vi "Display Text from JSON.vi"(5 "No Error on Empty Input String":bool, 7 "Alphabetical Sort Objects":bool, 8 "error in (no error)":errorcluster, 10 "Offset":i32, 11 "Input JSON":string) -> (0 "error out":errorcluster, 1 "Offset after first JSON Value":i32, 3 "Display Text":string)   [LabVIEW 2021, in "json.facade.lvlib"]
doc: "Reformate JSON as a more human-readable text string, for use in displays. The format is similar to YAML, but may not be fully compliant with that format."
uses:
  json.facade.lvlib
  jsontext/JSONtext.lvlib
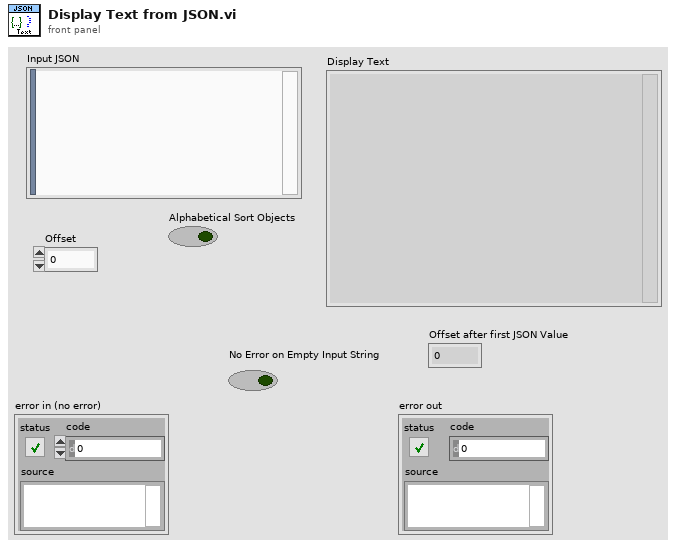
[diagram p1: front panel]
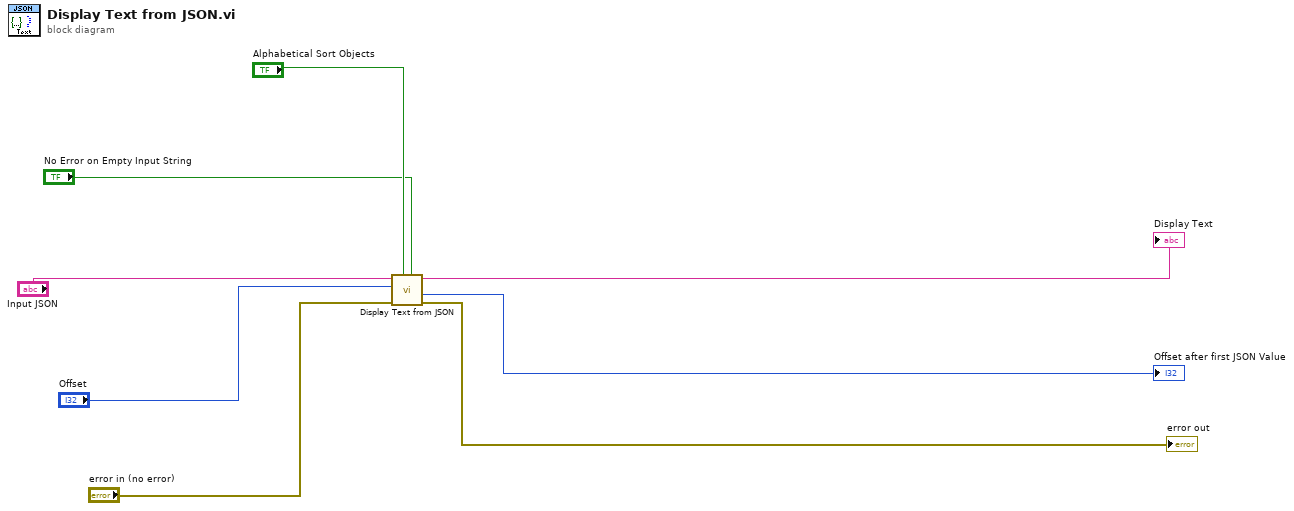
[diagram p0: block diagram]
diagram:
  n1 = call "Display Text from JSON.vi"("No Error on Empty Input String"="No Error on Empty Input String", "Alphabetical Sort Objects"="Alphabetical Sort Objects", "error in (no error)"="error in (no error)", "Offset"="Offset", "Input JSON"="Input JSON") -> ("error out"=→"error out":errorcluster, "Offset after first JSON Value"=→"Offset after first JSON Value":i32, "Display Text"=→"Display Text":string)  [unwired: 4 in]
